vi "PCResponse.vi"(11 "Array":string[](array[string])) -> (3 "Array 2":string[](array[string]))   [LabVIEW 2026]
uses:
  <vilib>/numeric/Random Number (Range) U64.vi
  <vilib>/numeric/sub_Random U32.vi
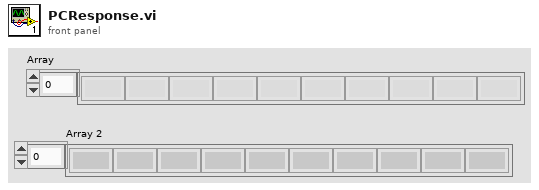
[diagram p1: front panel]
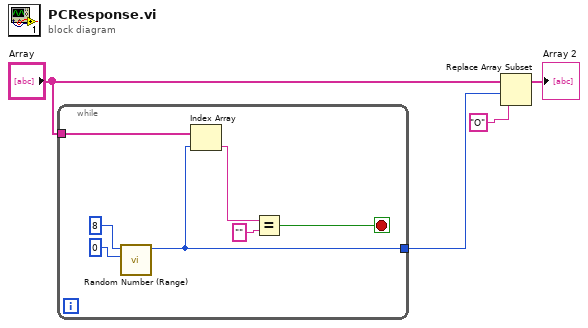
[diagram p0: block diagram]
diagram:
  n1 = while {
    tunnel: "Array" -> [w6]
    tunnel: [w5] -> w3
    stop <- w7 stop-if-true
    n2 = call-poly <vilib>:"Random Number (Range).vi"("lower bound (0)"=u64 0, "upper bound (100)"=u64 8) -> ("number"=w5:u64)  [unwired: 9 in]
    n3 = Index Array(array=w6, index=w5) -> (element=w9:string)
    n4 = Equal?(x=w9, y="") -> (x = y?=w7:bool)
  }
  n5 = Replace Array Subset(array="Array", new element="O" ("new element/subarray"), index=w3) -> (→"Array 2":string[])
